vi "Autonomous Independent.vi"() -> ()   [LabVIEW 2017]
doc: "This VI is called when autonomous begins, and will automatically be terminated when autonomous ends. You can carry out timed or sensor driven robot movement independently without needing to return to the caller."
uses:
  Arm Control/Arm Motor.ctl
  <vilib>/Rock Robotics/Network Tables/NT Read String.vi
  Robot Global Data.vi
  Pigeon IMU.ctl
panel:
  in  "error in":errorcluster
  # "Be sure to right-click and choose Data Operations>>Make Current Value default if you want to save the array values with the VI"
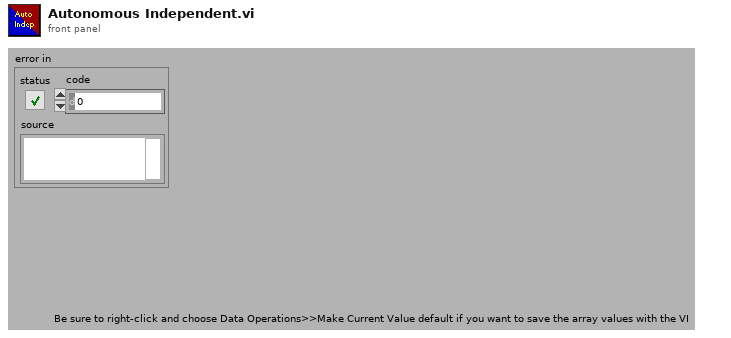
[diagram p1: front panel]
types:
  T1 = typedef "Arm Motor.ctl" = enum16{"Shoulder Motor", "Forearm Motor"}
  T2 = typedef "WPI_MotorControlDeviceRef.ctl" = cluster{"DeviceStatus":errorcluster, "Type":T3, "PWM":cluster{"PWM Channel":T4, "DeadBand":T5}, "CAN":cluster{"Device Number":u8, "SetOutput VI Ref":variant, "GetOutput VI Ref":variant, "Enable VI Ref":variant, "Disable VI Ref":variant, "Data":variant}, "Invert":bool, "DIO PWM":cluster{"PWM \"Enable\" Channel":T4, "DIOChannel":T6, "PWM Rate":dbl}}
  T3 = typedef "WPI_MotorControlType.ctl" = enum16{"PWM", "CAN", "DIO PWM"}
  T4 = typedef "FPGA_DIOPWMChannel.ctl" = enum8{"PWM 0", "PWM 1", "PWM 2", "PWM 3", "PWM 4", "PWM 5", "PWM 6", "PWM 7", "PWM 8", "PWM 9", "PWM MXP 0", "PWM MXP 1", "PWM MXP 2", "PWM MXP 3", "PWM MXP 4", "PWM MXP 5", "PWM MXP 6", "PWM MXP 7", "PWM MXP 8", "PWM MXP 9", "Invalid"}
  T5 = typedef "WPI_PWMDeadband.ctl" = cluster{"Name":string, "maxPositivePwm":i32, "minPositivePwm":i32, "centerPwm":i32, "maxNegativePwm":i32, "minNegativePwm":i32, "angularRange":u16}
  T6 = typedef "FPGA_DIOChannel.ctl" = enum8{"DIO 0", "DIO 1", "DIO 2", "DIO 3", "DIO 4", "DIO 5", "DIO 6", "DIO 7", "DIO 8", "DIO 9", "DIO MXP 0", "DIO MXP 1", "DIO MXP 2", "DIO MXP 3", "DIO MXP 4", "DIO MXP 5", "DIO MXP 6", "DIO MXP 7", "DIO MXP 8", "DIO MXP 9", "DIO MXP 10", "DIO MXP 11", "DIO MXP 12", "DIO MXP 13", "DIO MXP 14", "DIO MXP 15", "SPI Port CS1", "SPI Port CS2", "SPI Port CS3", "SPI Port MISO", "SPI Port MOSI", "Invalid"}
  T7 = typedef "Pigeon IMU.ctl" = enum16{"Pigeon IMU"}
  T8 = typedef "CTRE_PigeonIMU_DeviceRef.ctl" = cluster{"DeviceStatus":errorcluster, "Device Number":u8, "Type":T9, "Device ID":u32, "Handle":u64, "UsageFrame":u32, "Library Path":path}
  T9 = typedef "CTRE_PigeonIMU_ConnectionType.ctl" = u32
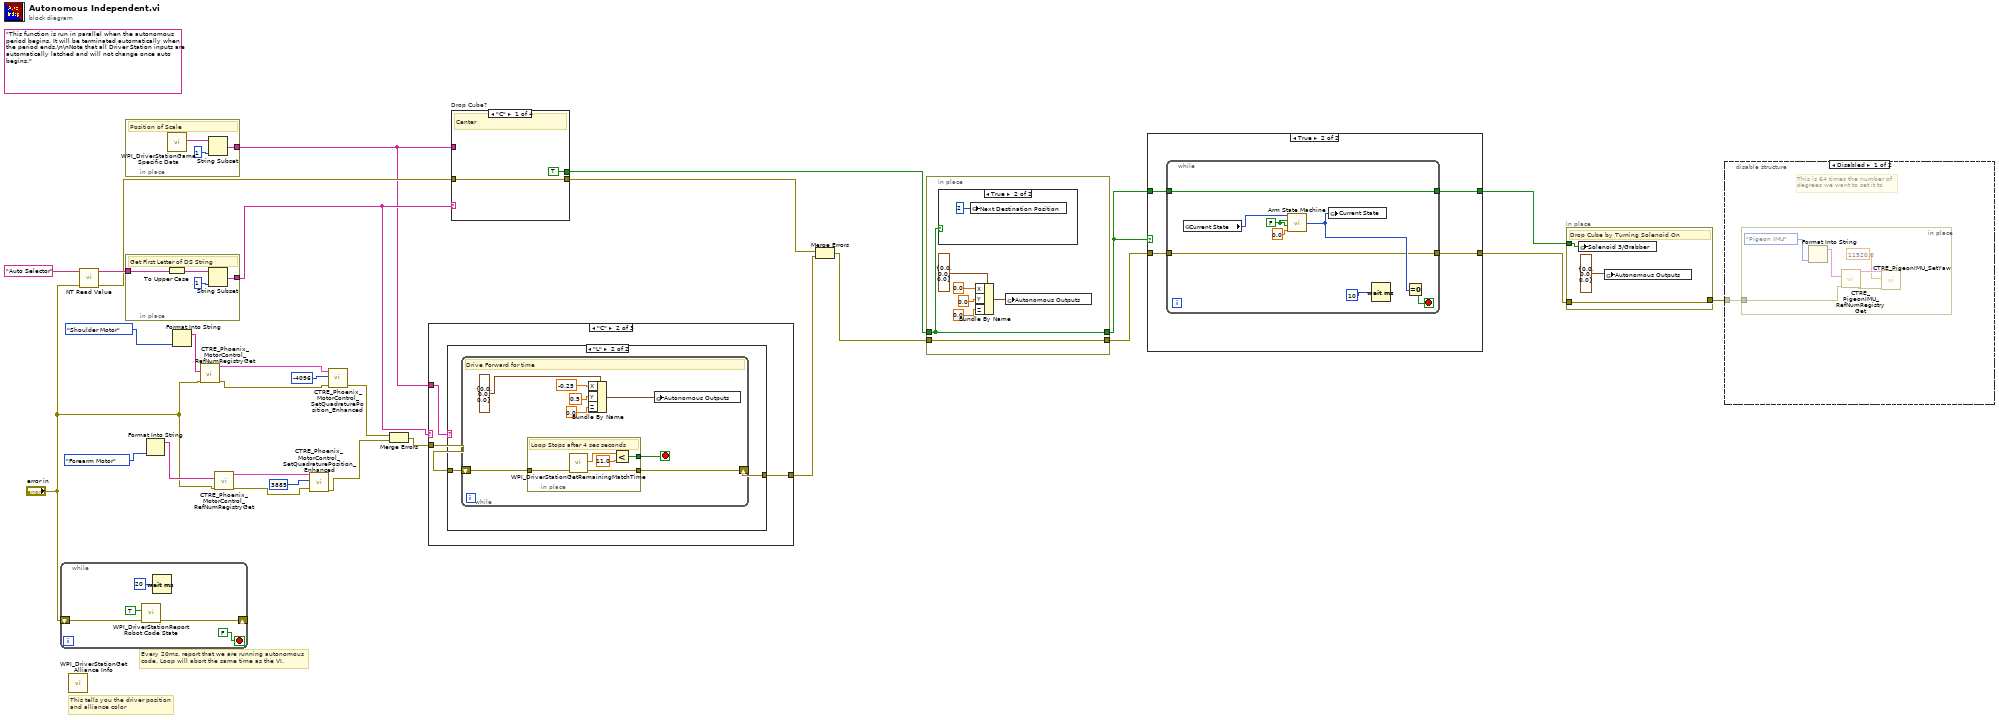
[diagram p0: block diagram]
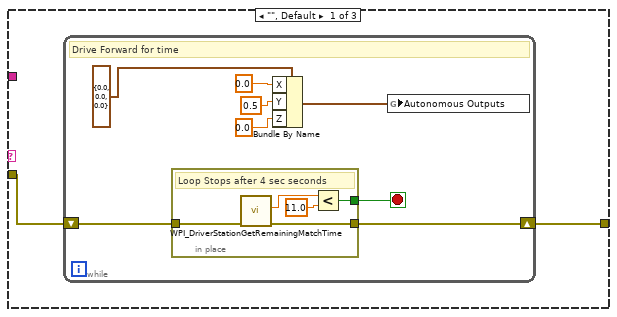
[diagram p3: hidden frame]
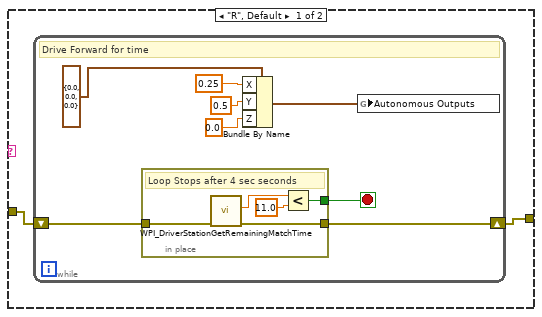
[diagram p4: hidden frame]
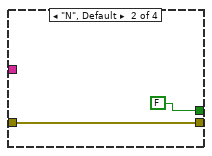
[diagram p8: hidden frame]
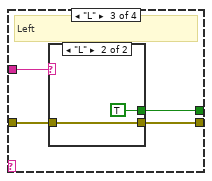
[diagram p9: hidden frame]
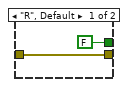
[diagram p10: hidden frame]
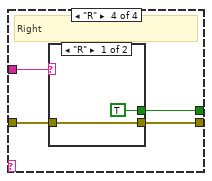
[diagram p11: hidden frame]
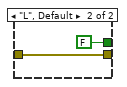
[diagram p12: hidden frame]
diagram:
  (unwired) "This function is run in parallel when the autonomous period begins. It will be terminated automatically when the period ends.\n\nNote that all Driver Station inputs are automatically latched and will not change once auto begins."
  # "Every 20ms, report that we are running autonomous\ncode. Loop will abort the same time as the VI."
  # "This tells you the driver position\nand alliance color"
  n1 = while {
    shift-right: [w29] -> _
    shift-left: "error in" -> [w30]
    stop <- FALSE stop-if-true
    n2 = call <vilib>:"WPI_DriverStationReport Robot Code State.vi"("error in (no error)"=w30, "Autonomous"=TRUE) -> ("error out"=w29:errorcluster)  [unwired: 9 in]
    n3 = Wait (ms)(milliseconds to wait=u32 20) -> ()  [unwired: 1 out]
  }
  n4 = call <vilib>:"WPI_DriverStationGet Alliance Info.vi"() -> ()  [unwired: 12 out]
  n5 = call-poly <vilib>:"NT Read Value.vi"("error in"="error in", "Name"="Auto Selector") -> ("error out"=w26:errorcluster, "String"=w27:string)  [unwired: 8 in]
  n6 = in-place {
    in-place-border: [w34] -> w3
    # "Position of Scale"
    n7 = call <vilib>:"WPI_DriverStationGame Specific Data.vi"() -> ("Game Specific Data"=w36:string)  [unwired: 11 in]
    n8 = String Subset(string=w36, length (rest)=1 ("length (rest)")) -> (substring=w34:string)  [unwired: 1 in]
  }
  n9 = in-place {
    in-place-border: w27 -> [w40]
    in-place-border: [w37] -> w4
    # "Get First Letter of DS String"
    n10 = To Upper Case(1:w40) -> (0:w39:string)
    n11 = String Subset(string=w39, length (rest)=1 ("length (rest)")) -> (substring=w37:string)  [unwired: 1 in]
  }
  n12 = Format Into String(Arm_Motor."Forearm Motor" ("Enum")) -> (resulting string=w11:string)  [unwired: 3 in, 1 out]
  n13 = Format Into String(Arm_Motor."Shoulder Motor" ("Enum")) -> (resulting string=w8:string)  [unwired: 3 in, 1 out]
  n14 = call "CTRE_Phoenix_MotorControl_RefNumRegistryGet.vi"("error in (no error)"="error in", "refnum name"=w8) -> ("error out"=w9:errorcluster, "PhoenixMotorControlDevRef"=w6:T2)  [unwired: 8 in]
  n15 = call "CTRE_Phoenix_MotorControl_RefNumRegistryGet.vi"("error in (no error)"="error in", "refnum name"=w11) -> ("error out"=w13:errorcluster, "PhoenixMotorControlDevRef"=w5:T2)  [unwired: 8 in]
  n16 = call <vilib>:"CTRE_Phoenix_MotorControl_SetQuadraturePosition_Enhanced.vi"("error in (no error)"=w13, "New Position"=3885, "PhoenixMotorControlDevRef"=w5) -> ("error out"=w15:errorcluster)  [unwired: 7 in, 1 out]
  n17 = call <vilib>:"CTRE_Phoenix_MotorControl_SetQuadraturePosition_Enhanced.vi"("error in (no error)"=w9, "New Position"=-4096, "PhoenixMotorControlDevRef"=w6) -> ("error out"=w16:errorcluster)  [unwired: 7 in, 1 out]
  n18 = Merge Errors(w16, w15) -> (w14:errorcluster)
  n19 = case shown="\"C\"" w4 {
    tunnel: [w42 w58 w89] -> w24
    tunnel: w14 -> [w41 w57 w89]
    tunnel: w3 -> [_ w56 _]
    frame "", Default {
      n20 = while {
        shift-right: [w43] -> w42
        shift-left: w41 -> [w44]
        stop <- w50 stop-if-true
        # "Drive Forward for time"
        n21 = in-place {
          in-place-border: [w54] -> w50
          in-place-border: w44 -> [w52]
          in-place-border: [w51] -> w43
          # "Loop Stops after 4 sec seconds"
          n22 = call <vilib>:"WPI_DriverStationGetRemainingMatchTime.vi"("error in (no error)"=w52) -> ("error out"=w51:errorcluster, "Match Time(s)"=w55:sgl)  [unwired: 9 in]
          n23 = Less?(x=w55, y=sgl 11.0) -> (x < y?=w54:bool)
        }
        n24 = Bundle By Name(cluster=cluster{"X":dbl, "Y":dbl, "Z":dbl} {"X"=0.0, "Y"=0.0, "Z"=0.0} ("Autonomous Outputs"), "X"=0.0, "Y"=0.5, "Z"=0.0) -> (w48:cluster{"X":dbl, "Y":dbl, "Z":dbl})
        n25 = global write "Robot Global Data.vi" "Autonomous Outputs"(w48) -> ()
      }
    }
    frame "C" {
      n26 = case shown="\"L\"" w56 {
        tunnel: [w59 w75] -> w58
        tunnel: w57 -> [w60 w74]
        frame "R", Default {
          n27 = while {
            shift-right: [w61] -> w59
            shift-left: w60 -> [w62]
            stop <- w68 stop-if-true
            # "Drive Forward for time"
            n28 = in-place {
              in-place-border: [w72] -> w68
              in-place-border: w62 -> [w70]
              in-place-border: [w69] -> w61
              # "Loop Stops after 4 sec seconds"
              n29 = call <vilib>:"WPI_DriverStationGetRemainingMatchTime.vi"("error in (no error)"=w70) -> ("error out"=w69:errorcluster, "Match Time(s)"=w73:sgl)  [unwired: 9 in]
              n30 = Less?(x=w73, y=sgl 11.0) -> (x < y?=w72:bool)
            }
            n31 = Bundle By Name(cluster=cluster{"X":dbl, "Y":dbl, "Z":dbl} {"X"=0.0, "Y"=0.0, "Z"=0.0} ("Autonomous Outputs"), "X"=0.25, "Y"=0.5, "Z"=0.0) -> (w66:cluster{"X":dbl, "Y":dbl, "Z":dbl})
            n32 = global write "Robot Global Data.vi" "Autonomous Outputs"(w66) -> ()
          }
        }
        frame "L" {
          n33 = while {
            shift-right: [w76] -> w75
            shift-left: w74 -> [w77]
            stop <- w83 stop-if-true
            # "Drive Forward for time"
            n34 = in-place {
              in-place-border: [w87] -> w83
              in-place-border: w77 -> [w85]
              in-place-border: [w84] -> w76
              # "Loop Stops after 4 sec seconds"
              n35 = call <vilib>:"WPI_DriverStationGetRemainingMatchTime.vi"("error in (no error)"=w85) -> ("error out"=w84:errorcluster, "Match Time(s)"=w88:sgl)  [unwired: 9 in]
              n36 = Less?(x=w88, y=sgl 11.0) -> (x < y?=w87:bool)
            }
            n37 = Bundle By Name(cluster=cluster{"X":dbl, "Y":dbl, "Z":dbl} {"X"=0.0, "Y"=0.0, "Z"=0.0} ("Autonomous Outputs"), "X"=-0.25, "Y"=0.5, "Z"=0.0) -> (w81:cluster{"X":dbl, "Y":dbl, "Z":dbl})
            n38 = global write "Robot Global Data.vi" "Autonomous Outputs"(w81) -> ()
          }
        }
      }
    }
    frame "N" {
    }
  }
  n39 = case "Drop Cube?" shown="\"C\"" w4 {
    tunnel: w3 -> [_ _ w97 w105]
    tunnel: [TRUE FALSE w96 w104] -> w22
    tunnel: w26 -> [w90 w92 w95 w103]
    tunnel: [w90 w92 w94 w102] -> w25
    frame "C" {
      # "Center"
    }
    frame "N", Default {
    }
    frame "L" {
      # "Left"
      n40 = case shown="\"L\"" w97 {
        tunnel: [FALSE TRUE] -> w96
        tunnel: w95 -> [w98 w100]
        tunnel: [w98 w100] -> w94
        frame "R", Default {
        }
        frame "L" {
        }
      }
    }
    frame "R" {
      # "Right"
      n41 = case shown="\"R\"" w105 {
        tunnel: [TRUE FALSE] -> w104
        tunnel: [w106 w108] -> w102
        tunnel: w103 -> [w106 w108]
        frame "R" {
        }
        frame "L", Default {
        }
      }
    }
  }
  n42 = Merge Errors(w25, w24) -> (w23:errorcluster)
  n43 = in-place {
    in-place-border: w23 -> [w116]
    in-place-border: [w116] -> w21
    in-place-border: [w115] -> w20
    in-place-border: w22 -> [w115]
    n44 = case shown="True" w115 {
      frame False {
      }
      frame True {
        n45 = global write "Robot Global Data.vi" "Next Destination Position"(2) -> ()
      }
    }
    n46 = Bundle By Name(cluster=cluster{"X":dbl, "Y":dbl, "Z":dbl} {"X"=0.0, "Y"=0.0, "Z"=0.0} ("Autonomous Outputs"), "X"=0.0, "Y"=0.0, "Z"=0.0) -> (w114:cluster{"X":dbl, "Y":dbl, "Z":dbl})
    n47 = global write "Robot Global Data.vi" "Autonomous Outputs"(w114) -> ()
  }
  n48 = case shown="True" w20 {
    tunnel: w20 -> [w119 w123]
    tunnel: [w119 w122] -> w19
    tunnel: w21 -> [w118 w121]
    tunnel: [w118 w120] -> w2
    frame False {
    }
    frame True {
      n49 = while {
        tunnel: w123 -> [w131]
        tunnel: [w131] -> w122
        tunnel: w121 -> [w124]
        tunnel: [w124] -> w120
        stop <- w126 stop-if-true
        w128 = FALSE
        n50 = global read "Robot Global Data.vi" "Current State"() -> (w129:i32)
        n51 = call "Arm State Machine.vi"("Delta Angle"=0.0, "Shoulder Control"=w128, "Forearm Control"=w128, "State"=w129) -> ("Next State"=w125:i32)
        n52 = global write "Robot Global Data.vi" "Current State"(w125) -> ()
        n53 = Wait (ms)(milliseconds to wait=10) -> ()  [unwired: 1 out]
        n54 = Equal To 0?(x=w125) -> (x = 0?=w126:bool)
      }
    }
  }
  n55 = in-place {
    in-place-border: w19 -> [w133]
    in-place-border: w2 -> [w132]
    in-place-border: [w132] -> w1
    # "Drop Cube by Turning Solenoid On"
    n56 = global write "Robot Global Data.vi" "Solenoid 3/Grabber"(w133) -> ()
    n57 = global write "Robot Global Data.vi" "Autonomous Outputs"(cluster{"X":dbl, "Y":dbl, "Z":dbl} {"X"=0.0, "Y"=0.0, "Z"=0.0} ("Autonomous Outputs")) -> ()
  }
  n58 = disable-structure shown="Disabled" {
    disable-tunnel: w1 -> [w135 _]
    frame Disabled {
      # "This is 64 times the number of \ndegrees we want to set it to"
      n59 = in-place {
        in-place-border: w135 -> [w136]
        n60 = Format Into String(Pigeon_IMU."Pigeon IMU") -> (resulting string=w140:string)  [unwired: 3 in, 1 out]
        n61 = call "CTRE_PigeonIMU_RefNumRegistryGet.vi"("error in (no error)"=w136, "refnum name"=w140) -> ("error out"=w137:errorcluster, "PigeonIMUDevRef"=w139:T8)  [unwired: 8 in]
        n62 = call <vilib>:"CTRE_PigeonIMU_SetYaw.vi"("error in (no error)"=w137, "Value"=11520.0, "PigeonIMUDevRef"=w139) -> ()  [unwired: 7 in, 2 out]
      }
    }
    frame Enabled {
    }
  }
